vi "ATF-monitor screen.vi"() -> ()   [LabVIEW 2022 SP3]
panel:
  out "E_STOP_L":bool
  out "GDC_L":bool
  out "MCU2_RST_L":bool
  out "MCU1_RST_L":bool
  out "E_STOP_A":bool
  out "GDC_A":bool
  out "MCU2_RST_A":bool
  out "MCU1_RST_A":bool
  in  "V_DC_L":dbl format="%#_g V"
  in  "V_CA_L":dbl format="%#_g V"
  in  "V_BC_L":dbl format="%#_g V"
  in  "V_AB_L":dbl format="%#_g V"
  in  "I_DC_L":dbl format="%#_g A"
  in  "I_C_L":dbl format="%#_g A"
  in  "I_B_L":dbl format="%#_g A"
  in  "I_A_L":dbl format="%#_g A"
  in  "I_DC_A":dbl format="%#_g A"
  in  "I_C_A":dbl format="%#_g A"
  in  "I_B_A":dbl format="%#_g A"
  in  "I_A_A":dbl format="%#_g A"
  in  "V_DC_A":dbl format="%#_g V"
  in  "V_CA_A":dbl format="%#_g V"
  in  "V_BC_A":dbl format="%#_g V"
  in  "V_AB_A":dbl format="%#_g V"
  in  "O_M_D_A":dbl format="%#_g K"
  in  "O_M_D_V":dbl format="%#_g K"
  in  "O_M_D_H":dbl format="%#_g K"
  in  "O_M_ND_A":dbl format="%#_g K"
  in  "O_M_ND_V":dbl format="%#_g K"
  in  "O_M_ND_H":dbl format="%#_g K"
  in  "O_P_B_A":dbl format="%#_g K"
  in  "O_P_B_V":dbl format="%#_g K"
  in  "O_P_B_H":dbl format="%#_g K"
  in  "O_P_A":dbl format="%#_g K"
  in  "O_P_V":dbl format="%#_g K"
  in  "O_P_H":dbl format="%#_g K"
  in  "F_M_D_A":dbl format="%#_g K"
  in  "F_M_D_V":dbl format="%#_g K"
  in  "F_M_D_H":dbl format="%#_g K"
  in  "F_M_ND_A":dbl format="%#_g K"
  in  "F_M_ND_V":dbl format="%#_g K"
  in  "F_M_ND_H":dbl format="%#_g K"
  in  "F_P_B_A":dbl format="%#_g K"
  in  "F_P_B_V":dbl format="%#_g K"
  in  "F_P_B_H":dbl format="%#_g K"
  in  "F_P_A":dbl format="%#_g K"
  in  "F_P_V":dbl format="%#_g K"
  in  "F_P_H":dbl format="%#_g K"
  in  "E_TC_ 5":dbl format="%#_g K"
  in  "E_TC_4":dbl format="%#_g K"
  in  "E_TC_3":dbl format="%#_g K"
  in  "E_TC_2":dbl format="%#_g K"
  in  "E_TC_1":dbl format="%#_g K"
  in  "I_TC_2":dbl format="%#_g K"
  in  "I_TC_1":dbl format="%#_g K"
  in  "TC_L_ND":dbl format="%#_g K"
  in  "TC_L_D":dbl format="%#_g K"
  in  "TC_L_C_2":dbl format="%#_g K"
  in  "TC_L_C_1":dbl format="%#_g K"
  in  "TC_A_ND":dbl format="%#_g K"
  in  "TC_A_D":dbl format="%#_g K"
  in  "TC_A_C_2":dbl format="%#_g K"
  out "C bottom open circuit - LOX":bool
  out "C top open circuit -LOX":bool
  out "B top open circuit - LOX":bool
  out "B Top Open circuit - LOX":bool
  out "A bottom open circuit -LOX":bool
  out "A Top Open circuit -LOX":bool
  out "C Bottom  Short Circuit - LOX":bool
  out "C top Short Circuit - LOX":bool
  out "B Bottom short circuit - LOX":bool
  out "B top Short circuit - LOX":bool
  out "A bottom short circuit - LOX":bool
  out "A top Short Circuit - LOX":bool
  out "Speed cmd & Response mismatch- LOX":bool
  out "Motor overload - LOX":bool
  out "Over temperature - LOX":bool
  out "Over speed - LOX":bool
  out "C Phase Short circuit - LOX":bool
  out "C Phase open circuit -LOX":bool
  out "B Phase Short circuit - LOX":bool
  out "B Phase open circuit-LOX":bool
  out "A phase short circuit-LOX":bool
  out "A Phase open circuit -LOX":bool
  out "C bottom open circuit - ATF":bool
  out "C top open circuit -ATF":bool
  out "B top open circuit - ATF":bool
  out "B Top Open circuit - ATF":bool
  out "A bottom open circuit -ATF":bool
  out "A Top Open circuit -ATF":bool
  out "C Bottom  Short Circuit - ATF":bool
  out "C top Short Circuit - ATF":bool
  out "B Bottom short circuit - ATF":bool
  out "B top Short circuit - ATF":bool
  out "A bottom short circuit - ATF":bool
  out "A top Short Circuit - ATF":bool
  out "Speed cmd & Response mismatch- ATF":bool
  out "Motor overload - ATF":bool
  out "Over temperature - ATF":bool
  out "Over speed - ATF":bool
  out "C Phase Short circuit - ATF":bool
  out "C Phase open circuit -ATF":bool
  out "B Phase Short circuit - ATF":bool
  out "B Phase open circuit-ATF":bool
  out "A phase short circuit-ATF":bool
  out "A Phase open circuit -ATF":bool
  out "Master - Slave Failure":bool
  out "Over Power Detection":bool
  out "Over Current Detection":bool
  out "Over Voltage Detection":bool
  out "Power fail Status":bool
  out "Alarm":bool
  out "PPSU Health":bool
  out "No. of Slave Devices":dbl
  in  "Terminal Power":dbl format="%#_g W"
  in  "Terminal Current":dbl format="%#_g A"
  in  "Terminal Voltage":dbl format="%#_g V"
  in  "EXIT":bool
  # "VERSION NUMBER : 1.2"
  # "SeCrTs- MONITORING GUI 1"
  # "RELEASE DATE :10/06/2024"
  # "Critical Parameters"
  # "PPSU Responses & Feedback"
  # "Thermal Data"
  # "Drive LOX Critical Parameters"
  # "Drive ATF Critical Parameters"
  # "Gate driver"
  # "MCU2_RST_L"
  # "MCU1_RST_L"
  # "MCU2_RST_A"
  # "MCU1_RST_A"
  # "E_STOP_L"
  # "GDC_L"
  # "E_STOP_A"
  # "GDC_A"
  # "Vibration  Data"
  # "Drive ATF Fault Status"
  # "Drive LOX Fault Status"
  # "A-Phase top\nMOSFET Open circuit"
  # "A-Phase top MOSFET Short circuit"
  # "A-Phase top\nMOSFET Open circuit"
  # "A-Phase top MOSFET Short circuit"
  # "A-Phase open circuit"
  # "A-Phase open circuit"
  # "A-Phase Short circuit"
  # "A-Phase Short circuit"
  # "A-Phase bottom MOSFET Open circuit"
  # "A-Phase bottom MOSFET Open circuit"
  # "A-Phase bottom MOSFET Short circuit"
  # "A-Phase bottom MOSFET Short circuit"
  # "B-Phase Open circuit"
  # "B-Phase Open circuit"
  # "Pressure Data"
  # "B-Phase top MOSFET Short circuit"
  # "B-Phase top MOSFET Short circuit"
  # "B-Phase Short circuit"
  # "B-Phase Short circuit"
  # "B-Phase top MOSFET Open circuit"
  # "B-Phase top MOSFET Open circuit"
  # "C-Phase Open circuit"
  # "C-Phase Open circuit"
  # "B-Phase Bottom MOSFET Short circuit"
  # "B-Phase Bottom MOSFET Short circuit"
  # "B-Phase Bottom MOSFET Open circuit"
  # "B-Phase Bottom MOSFET Open circuit"
  # "C-Phase Short circuit"
  # "C-Phase Short circuit"
  # "C-Phase top MOSFET Open circuit"
  # "C-Phase top MOSFET Open circuit"
  # "C-Phase top MOSFET Short circuit"
  # "Over speed"
  # "C-Phase top MOSFET Short circuit"
  # "Over speed"
  # "Critical Data"
  # "Over Temperature"
  # "Over Temperature"
  # "C-Phase Bottom MOSFET Open circuit"
  # "C-Phase Bottom MOSFET Short circuit"
  # "C-Phase Bottom MOSFET Open circuit"
  # "C-Phase Bottom MOSFET Short circuit"
  # "Motor Overload"
  # "Motor Overload"
  # "Speed Command & response mismatch"
  # "Speed Command & response mismatch"
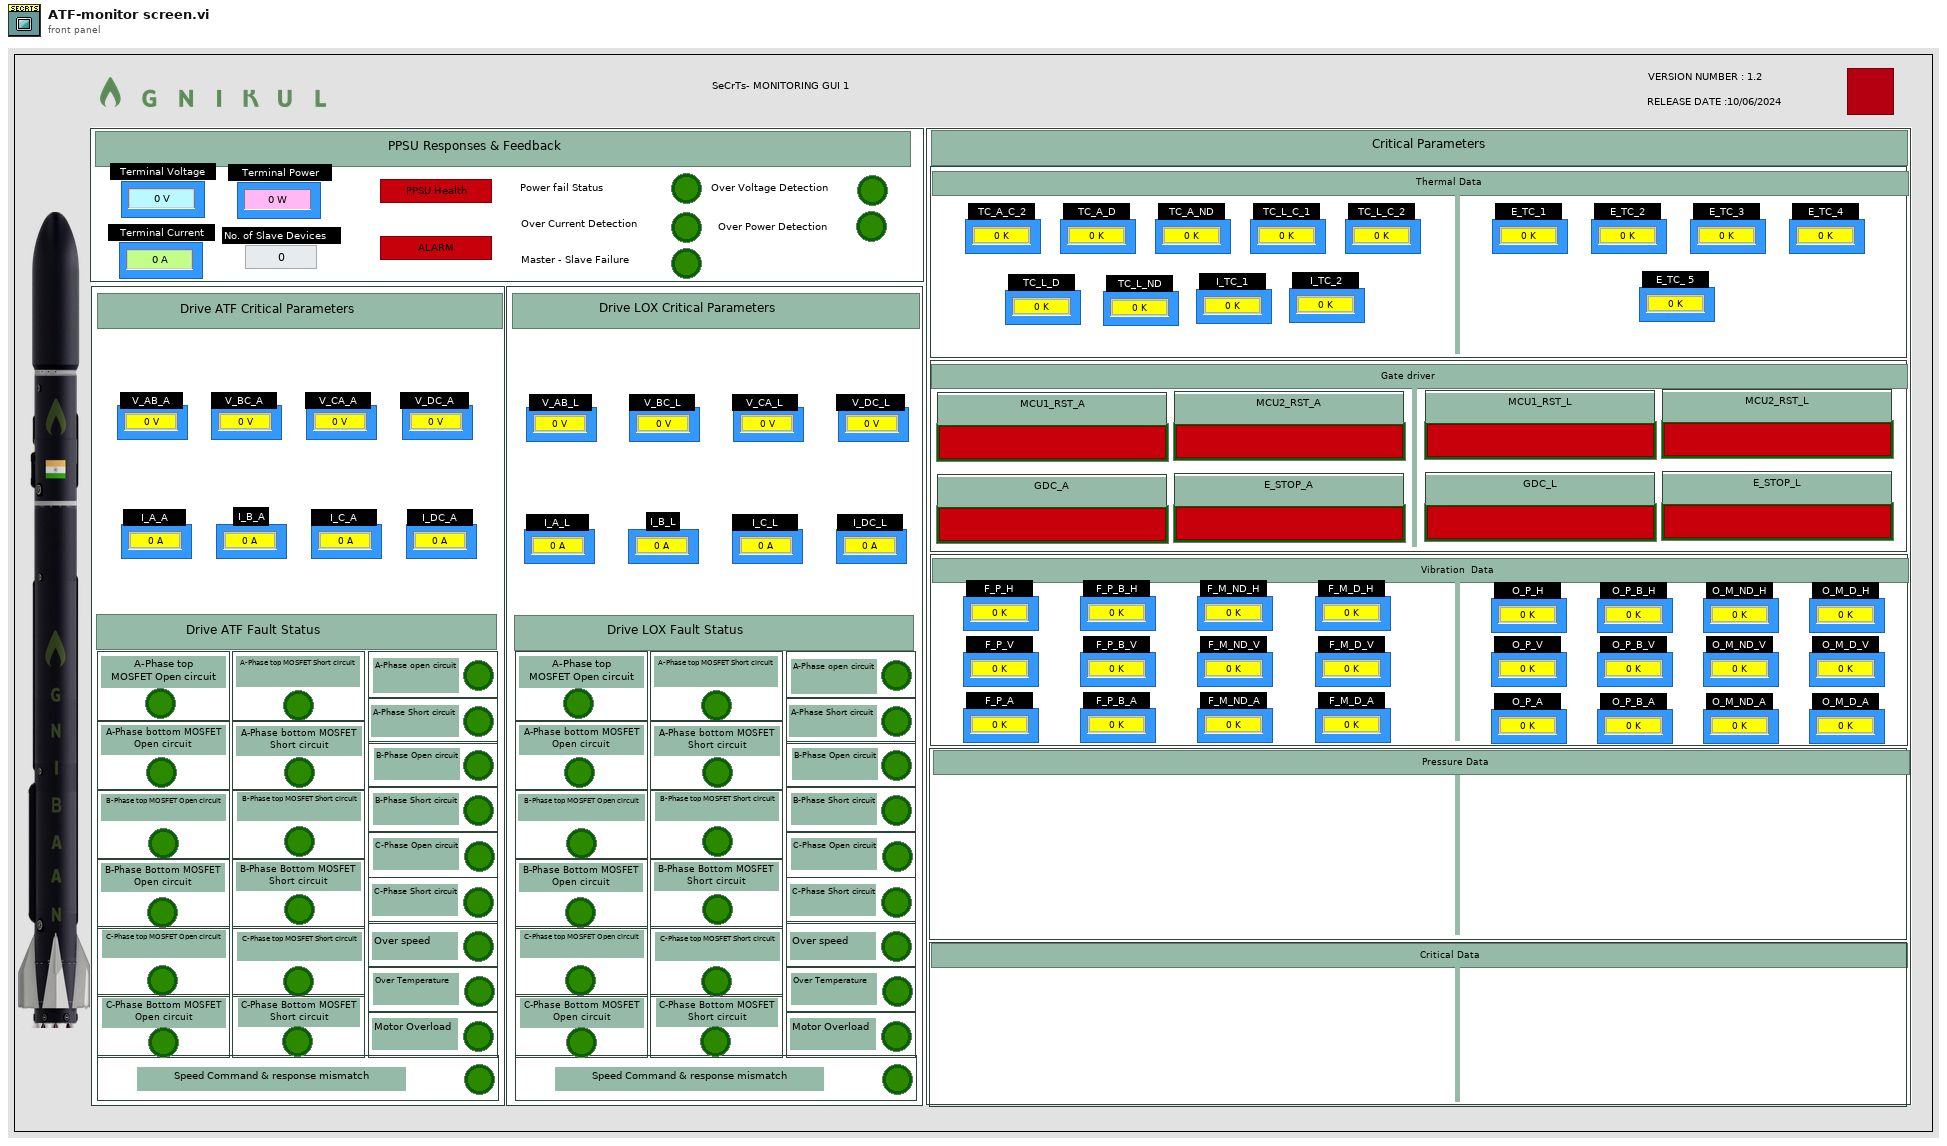
[diagram p1: front panel]
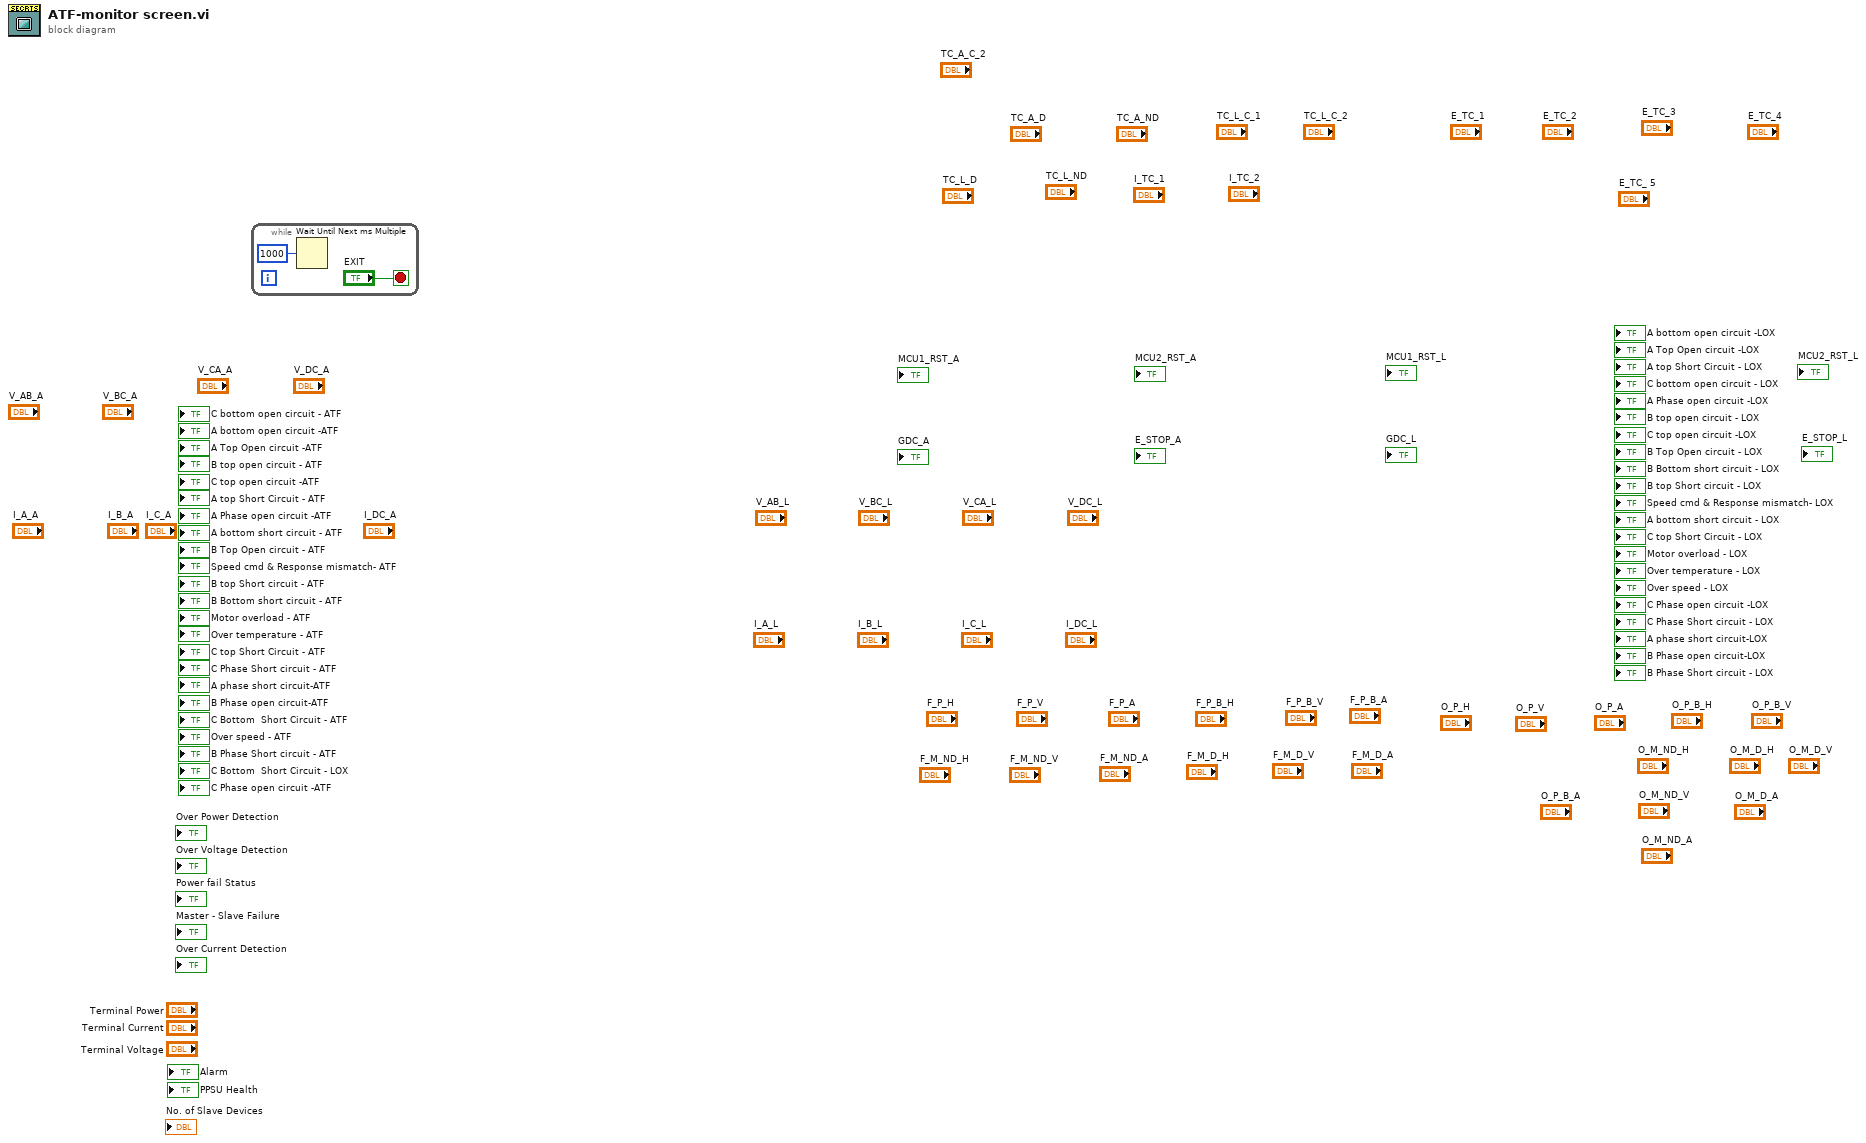
[diagram p0: block diagram]
diagram:
  n1 = while {
    stop <- "EXIT" stop-if-true
    n2 = Wait Until Next ms Multiple(millisecond multiple=u32 1000) -> ()  [unwired: 1 out]
  }
